vi "GetTeamData4Edit.vi"(10 "Team #":string) -> (0 "Pictures":string[](array[string]), 1 "Data":string[](array[string]), 2 "Location":string, 3 "Name":string)   [LabVIEW 2017]
uses:
  <vilib>/Utility/config.llb/Read Key (String).vi
  <vilib>/Utility/config.llb/NI_LVConfig.lvlib
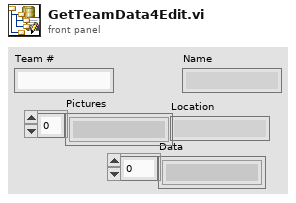
[diagram p1: front panel]
types:
  T1 = typedef "NI_LVConfig.lvlib/Config Data RefNum.ctl" = refnum<k1>
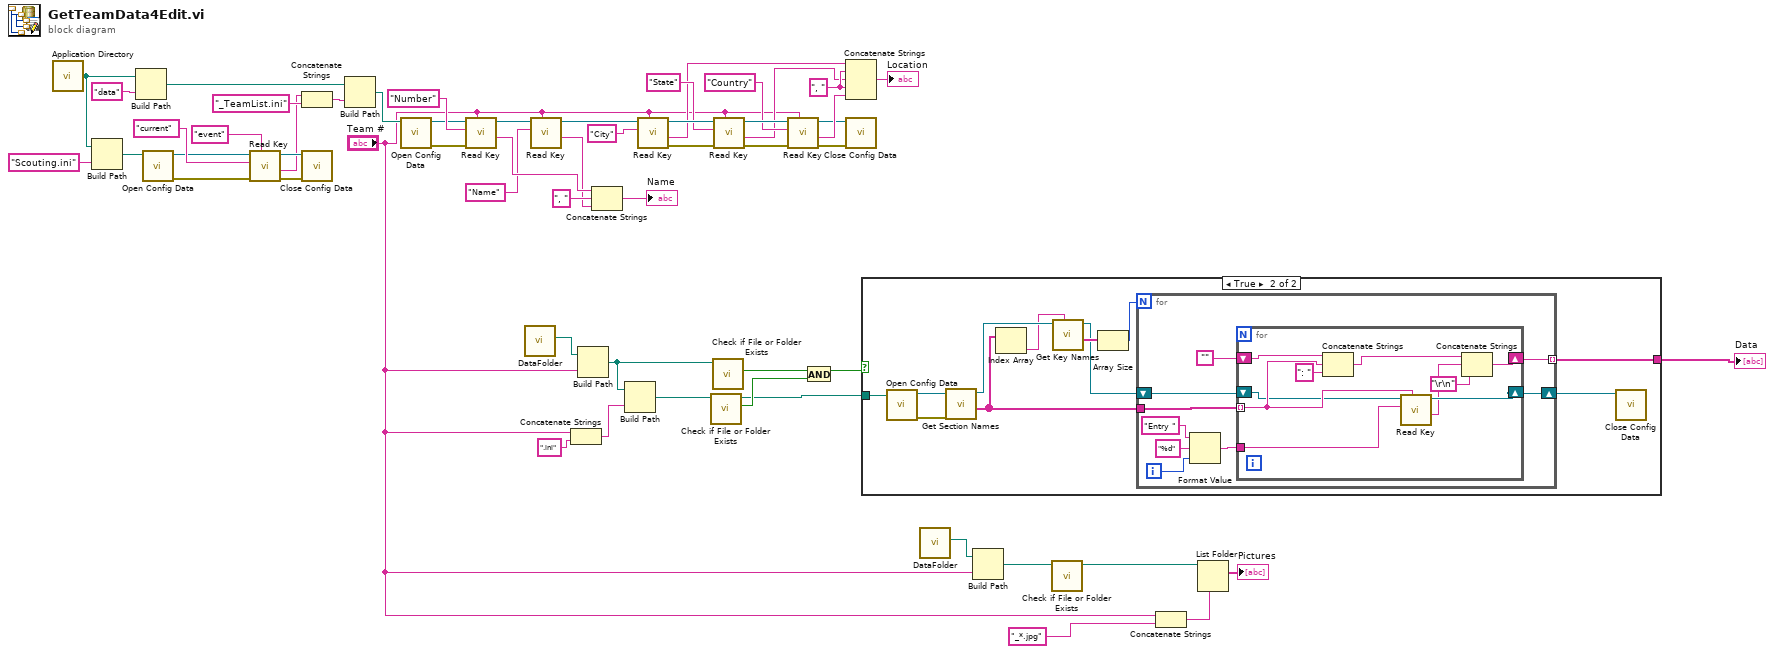
[diagram p0: block diagram]
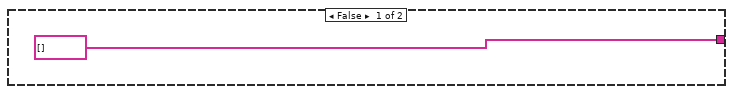
[diagram p2: hidden frame]
diagram:
  w24 = ", " ("string")
  n1 = call <vilib>:"Application Directory.vi"() -> ("Application Directory"=w45:path)
  n2 = Build Path(base path=w45, name or relative path="Scouting.ini") -> (appended path=w38:path)
  n3 = Build Path(base path=w45, name or relative path="data") -> (appended path=w40:path)
  n4 = call <vilib>:"Open Config Data.vi"("configuration file path"=w38) -> ("error out"=w32:errorcluster, "refnum"=w33:T1)  [unwired: 8 in, 1 out]
  n5 = call-poly <vilib>:"Read Key.vi"("section"="event" ("key"), "error in (no error)"=w32, "key"="current" ("section"), "refnum"=w33) -> ("error out"=w34:errorcluster, "value"=w25:string, "refnum out"=w35:T1)  [unwired: 4 in, 1 out]
  n6 = Concatenate Strings(w25, "_TeamList.ini" ("string")) -> (w41:string)
  n7 = call <vilib>:"Close Config Data.vi"("error in (no error)"=w34, "refnum"=w35) -> ()  [unwired: 8 in, 2 out]
  n8 = Build Path(base path=w40, name or relative path=w41) -> (appended path=w44:path)
  n9 = call <vilib>:"Open Config Data.vi"("configuration file path"=w44) -> ("error out"=w46:errorcluster, "refnum"=w47:T1)  [unwired: 8 in, 1 out]
  n10 = call-poly <vilib>:"Read Key.vi"("section"="Team #", "error in (no error)"=w46, "key"="Number", "refnum"=w47) -> ("value"=w52:string, "refnum out"=w49:T1)  [unwired: 4 in, 2 out]
  n11 = call "DataFolder.vi"() -> ("appended path"=w17:path)  [unwired: 11 in]
  n12 = call-poly <vilib>:"Read Key.vi"("section"="Team #", "key"="Name", "refnum"=w49) -> ("value"=w51:string, "refnum out"=w55:T1)  [unwired: 5 in, 2 out]
  n13 = Concatenate Strings("Team #", ".ini" ("format string")) -> (w14:string)
  n14 = Build Path(base path=w17, name or relative path="Team #") -> (appended path=w13:path)
  n15 = Concatenate Strings(w52, ", " ("string"), w51) -> (→"Name":string)
  n16 = Build Path(base path=w13, name or relative path=w14) -> (appended path=w12:path)
  n17 = call-poly <vilib>:"Read Key.vi"("section"="Team #", "key"="City", "refnum"=w55) -> ("error out"=w30:errorcluster, "value"=w23:string, "refnum out"=w31:T1)  [unwired: 5 in, 1 out]
  n18 = call <vilib>:"Check if File or Folder Exists.vi"("path"=w12) -> ("file or folder exists?"=w10:bool, "dup path"=w9:path)  [unwired: 8 in, 1 out]
  n19 = call <vilib>:"Check if File or Folder Exists.vi"("path"=w13) -> ("file or folder exists?"=w16:bool)  [unwired: 8 in, 2 out]
  n20 = call-poly <vilib>:"Read Key.vi"("section"="Team #", "error in (no error)"=w30, "key"="State", "refnum"=w31) -> ("error out"=w28:errorcluster, "value"=w22:string, "refnum out"=w29:T1)  [unwired: 4 in, 1 out]
  n21 = call-poly <vilib>:"Read Key.vi"("section"="Team #", "error in (no error)"=w28, "key"="Country", "refnum"=w29) -> ("error out"=w19:errorcluster, "value"=w21:string, "refnum out"=w18:T1)  [unwired: 4 in, 1 out]
  n22 = And(x=w16, y=w10) -> (x .and. y?=w11:bool)
  n23 = Concatenate Strings(w23, w24, w22, w24, w21) -> (→"Location":string)
  n24 = call <vilib>:"Close Config Data.vi"("error in (no error)"=w19, "refnum"=w18) -> ()  [unwired: 8 in, 2 out]
  n25 = case shown="True" w11 {
    tunnel: [string[] [] ("key") w58] -> w1
    tunnel: w9 -> [_ w68]
    frame False {
    }
    frame True {
      n26 = call <vilib>:"Open Config Data.vi"("configuration file path"=w68) -> ("error out"=w67:errorcluster, "refnum"=w66:T1)  [unwired: 8 in, 1 out]
      n27 = call <vilib>:"Get Section Names.vi"("error in (no error)"=w67, "refnum"=w66) -> ("section names"=w62:string[], "refnum out"=w64:T1)  [unwired: 7 in, 1 out]
      n28 = Index Array(array=w62) -> (element=w63:string)  [unwired: 1 in]
      n29 = call <vilib>:"Get Key Names.vi"("section"=w63, "refnum"=w64) -> ("key names"=w61:string[], "refnum out"=w60:T1)  [unwired: 6 in, 2 out]
      n30 = Array Size(array=w61) -> (size(s)=w59:i32)
      n31 = for {
        N: w59 -> [_]
        tunnel: w62 -> [w76]
        shift-right: [w77] -> w65
        shift-left: w60 -> [w74]
        tunnel: [w73] -> w58 mode=indexing
        i -> [w70]
        n32 = Format Value(string ("")="Entry ", format string="%d", value (0)=w70) -> (output string=w69:string)
        n33 = for {
          tunnel: w76 -> [w85] mode=indexing
          shift-right: [w87] -> w77
          shift-left: w74 -> [w84]
          shift-right: [w81] -> w73
          shift-left: "" -> [w82]
          tunnel: w69 -> [w79]
          n34 = Concatenate Strings(w82, w85, ": " ("string")) -> (w83:string)
          n35 = call-poly <vilib>:"Read Key.vi"("section"=w85, "key"=w79, "refnum"=w84) -> ("value"=w80:string, "refnum out"=w87:T1)  [unwired: 5 in, 2 out]
          n36 = Concatenate Strings(w83, w80, "\r\n") -> (w81:string)
        }
      }
      n37 = call <vilib>:"Close Config Data.vi"("refnum"=w65) -> ()  [unwired: 9 in, 2 out]
    }
  }
  "Data" <- w1
  n38 = call "DataFolder.vi"() -> ("appended path"=w8:path)  [unwired: 11 in]
  n39 = Build Path(base path=w8, name or relative path="Team #") -> (appended path=w7:path)
  n40 = call <vilib>:"Check if File or Folder Exists.vi"("path"=w7) -> ("dup path"=w4:path)  [unwired: 8 in, 2 out]
  n41 = Concatenate Strings("Team #", "_*.jpg" ("string")) -> (w5:string)
  n42 = List Folder(path=w4, pattern=w5) -> (filenames=→"Pictures":string[])  [unwired: 2 in, 3 out]
